vi "3-3 콜라자판기.vi"() -> ()   [LabVIEW 2014]
panel:
  in  "동전":cluster{"500":bool, "100":bool}
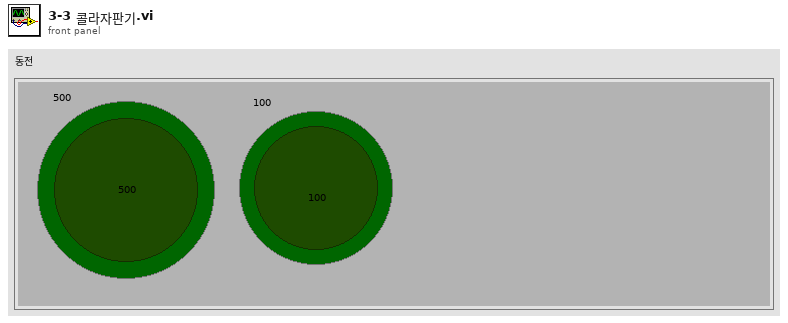
[diagram p1: front panel]
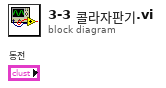
[diagram p0: block diagram]
diagram:
